vi "Display Entry.vi"(0 "Array of strings.":string[](array[string])) -> (1 "Single string.":string, 2 "Array of string lengths.":sgl[](array[numeric]) format="%.2f")   [LabVIEW 2010]
doc: "Convert the array of strings to a single string with end of line markers between the array entries. Construct an array consisting of the lengths of the strings in the srray of strings."
panel:
  # "Inputs:"
  # "Outputs:"
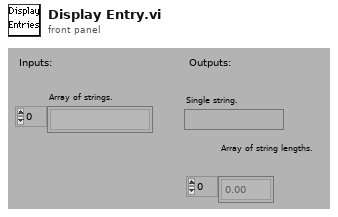
[diagram p1: front panel]
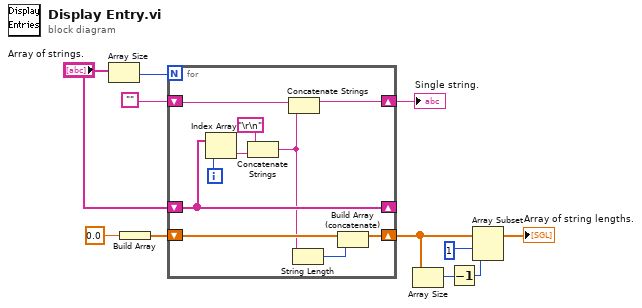
[diagram p0: block diagram]
diagram:
  n1 = Array Size(array="Array of strings.") -> (size(s)=w11:i32)
  n2 = Build Array(sgl 0.0) -> (w8:sgl[])
  n3 = for {
    N: w11 -> [_]
    shift-right: [w20] -> w1
    shift-left: "" -> [w21]
    shift-right: [w18] -> _
    shift-left: "Array of strings." -> [w18]
    shift-right: [w16] -> w6
    shift-left: w8 -> [w17]
    i -> [w19]
    n4 = Index Array(array=w18, index=w19) -> (element=w13:string)
    n5 = Concatenate Strings("\r\n", w13) -> (w14:string)
    n6 = Concatenate Strings(w21, w14) -> (w20:string)
    n7 = String Length(string=w14) -> (length=w15:i32)
    n8 = Build Array (concatenate)(w17, w15) -> (w16:sgl[])
  }
  "Single string." <- w1
  n9 = Array Size(array=w6) -> (size(s)=w5:i32)
  n10 = Decrement(x=w5) -> (x-1=w4:i32)
  n11 = Array Subset(array=w6, index=1, length=w4) -> (→"Array of string lengths.":sgl[])
